vi "OPO_save_points.vi"(3 "error in (no error)":errorcluster, 4 "Delay List":string[][](array[string]), 5 "file path (dialog if empty)":path) -> (0 "error out":errorcluster)   [LabVIEW 2019]
doc: "Saves out as a csv file the delay list"
uses:
  <vilib>/Utility/file.llb/Write Delimited Spreadsheet (string).vi
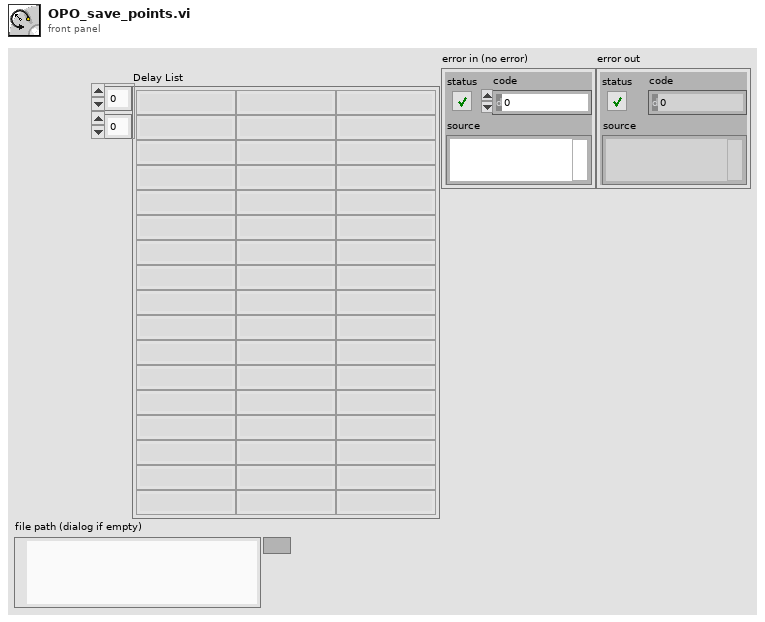
[diagram p1: front panel]
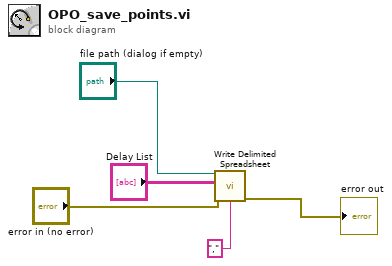
[diagram p0: block diagram]
diagram:
  n1 = call-poly <vilib>:"Write Delimited Spreadsheet.vi"("file path (dialog if empty)"="file path (dialog if empty)", "2D data"="Delay List", "error in (no error)"="error in (no error)", "delimiter (\\t)"="," ("delimiter (\\t)")) -> ("error out"=→"error out":errorcluster)  [unwired: 10 in, 1 out]
